vi "Exemple_Metrics_V_Measure_Score.vi"() -> ()   [LabVIEW 2020]
uses:
  Objet/3 - Model selection and evaluation/3.3 - Metrics and scoring/v_measure_score/V_Measure_Score.vi
panel:
  out "Score":string
  out "error out":errorcluster caption="sortie d'erreur"
  in  "v_measure_score":cluster{"beta":dbl}={"beta"=1.0}
  in  "error in (no error)":errorcluster caption="entrée d'erreur (pas d'erreur)"
  in  "labels_pred":string[][](array[string])=[["0"], ["0"], ["1"], ["1"]]
  in  "labels_true":string[][](array[string])=[["0"], ["0"], ["1"], ["2"]]
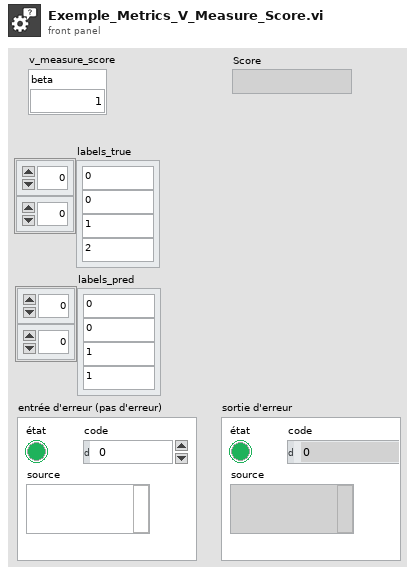
[diagram p1: front panel]
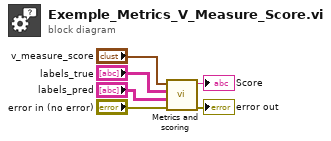
[diagram p0: block diagram]
diagram:
  n1 = call-poly "Metrics and scoring.vi"("error in (no error)"="error in (no error)", "labels_pred"="labels_pred", "labels_true"="labels_true", "v_measure_score"="v_measure_score") -> ("error out"=→"error out":errorcluster, "Score"=→"Score":string)  [unwired: 6 in]
